vi "Host - Testscreen Queue Driver.vi"(6 "timeout(ms)":i32=-1, 7 "Cases":T1, 8 "error in (no error)":errorcluster, 10 "Element In":cluster{"Data":variant, "Enum":T2}={"Data"=variant, "Enum"=enum."Update Test Results"}) -> (0 "error out":errorcluster, 2 "Element Out":cluster{"Data":variant, "Enum":T2}={"Data"=variant, "Enum"=enum."Update Test Results"}, 3 "queue out":refnum<queue>)   [LabVIEW 2017]
uses:
  TCP/TCP Host/Controls/Control - Testscreen.ctl
  TCP/TCP Host/Controls/Host- Queue States.ctl
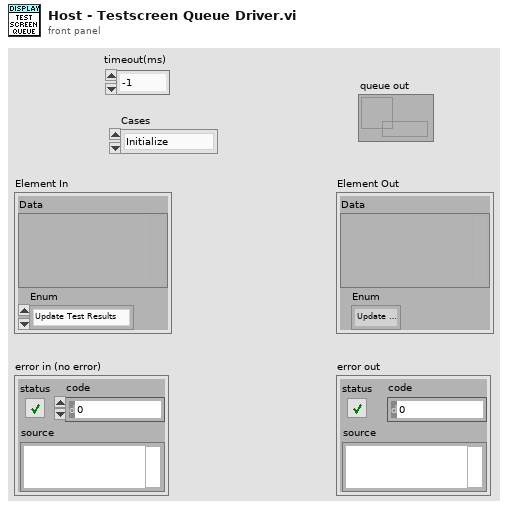
[diagram p1: front panel]
types:
  T1 = typedef "Host- Queue States.ctl" = enum16{"Initialize", "Enqueue", "Enqueue Priority", "Dequeue", "Flush", "Destroy"}
  T2 = typedef "Control - Testscreen.ctl" = enum16{"No Event", "Init", "Download Files", "Test Running", "Update Test Results", "Machine Unhealthy", "Autotest Started", "Test Aborted", "Sequence Complete", "Update Sensor Data", "Log File Available", "Machine Mode", "Aux Logging Started", "Aux File Saved", "Get PID Values", "View Report", "Exit", "Wait", "Abort", "Copy Log File", "Generate Alarm", "Send Test Details"}
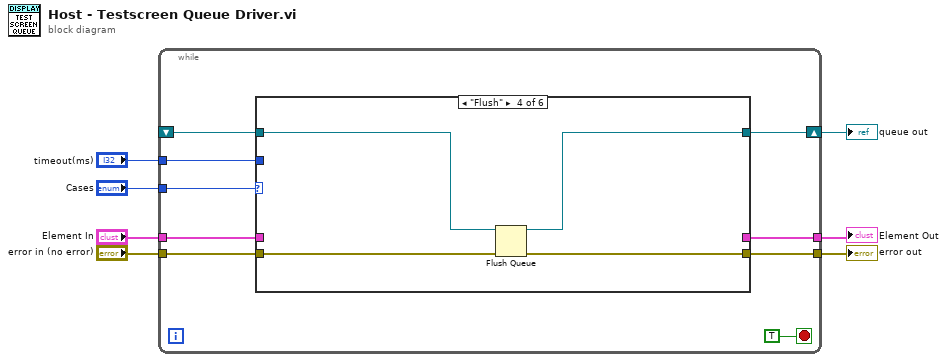
[diagram p0: block diagram]
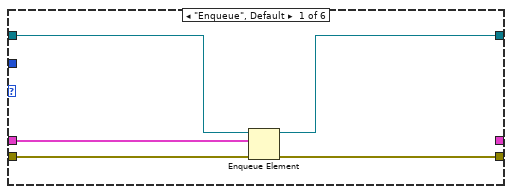
[diagram p2: hidden frame]
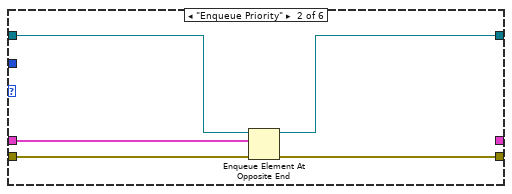
[diagram p3: hidden frame]
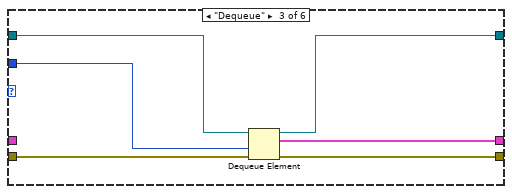
[diagram p4: hidden frame]
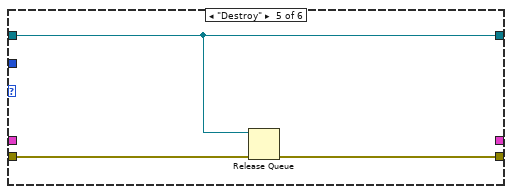
[diagram p5: hidden frame]
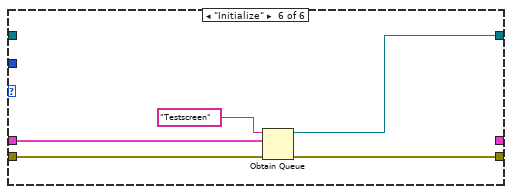
[diagram p6: hidden frame]
diagram:
  n1 = while {
    shift-right: [w15] -> w1
    shift-left: _ -> [w13]
    tunnel: "Cases" -> [w14]
    tunnel: "error in (no error)" -> [w12]
    tunnel: [w11] -> w5
    tunnel: "Element In" -> [w10]
    tunnel: [w9] -> w3
    tunnel: "timeout(ms)" -> [w8]
    stop <- TRUE stop-if-true
    n2 = case shown="\"Flush\"" w14 {
      tunnel: [w18 w23 w29 w33 w37 w43] -> w15
      tunnel: w13 -> [w19 w24 w30 w34 w37 _]
      tunnel: w12 -> [w21 w26 w32 w36 w39 w42]
      tunnel: [w20 w25 w31 w35 w38 w41] -> w11
      tunnel: w10 -> [w17 w22 _ _ _ w40]
      tunnel: [_ _ w28 _ _ _] -> w9
      tunnel: w8 -> [_ _ w27 _ _ _]
      frame "Enqueue", Default {
        n3 = Enqueue Element(queue=w19, element=w17, error in (no error)=w21) -> (queue out=w18:refnum<queue>, error out=w20:errorcluster)  [unwired: 1 in, 1 out]
      }
      frame "Enqueue Priority" {
        n4 = Enqueue Element At Opposite End(queue=w24, element=w22, error in (no error)=w26) -> (queue out=w23:refnum<queue>, error out=w25:errorcluster)  [unwired: 1 in, 1 out]
      }
      frame "Dequeue" {
        n5 = Dequeue Element(queue=w30, timeout in ms (-1)=w27, error in (no error)=w32) -> (queue out=w29:refnum<queue>, element=w28:cluster{"Data":variant, "Enum":T2}, error out=w31:errorcluster)  [unwired: 1 out]
      }
      frame "Flush" {
        n6 = Flush Queue(queue=w34, error in (no error)=w36) -> (queue out=w33:refnum<queue>, error out=w35:errorcluster)  [unwired: 1 out]
      }
      frame "Destroy" {
        n7 = Release Queue(queue=w37, error in (no error)=w39) -> (error out=w38:errorcluster)  [unwired: 1 in, 2 out]
      }
      frame "Initialize" {
        n8 = Obtain Queue(name (unnamed)="Testscreen", element data type=w40, error in (no error)=w42) -> (queue out=w43:refnum<queue>, error out=w41:errorcluster)  [unwired: 2 in, 1 out]
      }
    }
  }
  "error out" <- w5
  "queue out" <- w1
  "Element Out" <- w3
